vi "TestVI_TakeData.vi"() -> ()   [LabVIEW 2020]
uses:
  D:/Programs/Fatima/Lightfield-LabVIEW Automation/lightfield-automation-labview/TCube_motion/Kinesis/Thorlabs.MotionControl.Controls.dll
  Kinesis/Thorlabs.MotionControl.Controls.dll
panel:
  in  "Take data":bool
  in  "TOTAL STOP":bool
  out "Data":T1(array[cluster])
  out "ROI 1, Frame 1, Row 1":dbl[](graph)
  out "Intensity Graph":dbl[][](graph)
  in  "max":i32
  in  "min":i32
  in  "Start position X":dbl
  in  "Start position Y":dbl
  in  "Step Size Y":dbl
  in  "Step Size X":dbl
  in  "TotalSteps X":i32
  in  "TotalSteps Y":i32
  in  "SerialNumber X":string="83819717"
  in  "TCubeDCServoControl X":refnum<k24>(container)
  in  "SerialNumber Y":string="83817852"
  in  "TCubeDCServoControl Y":refnum<k24>(container)
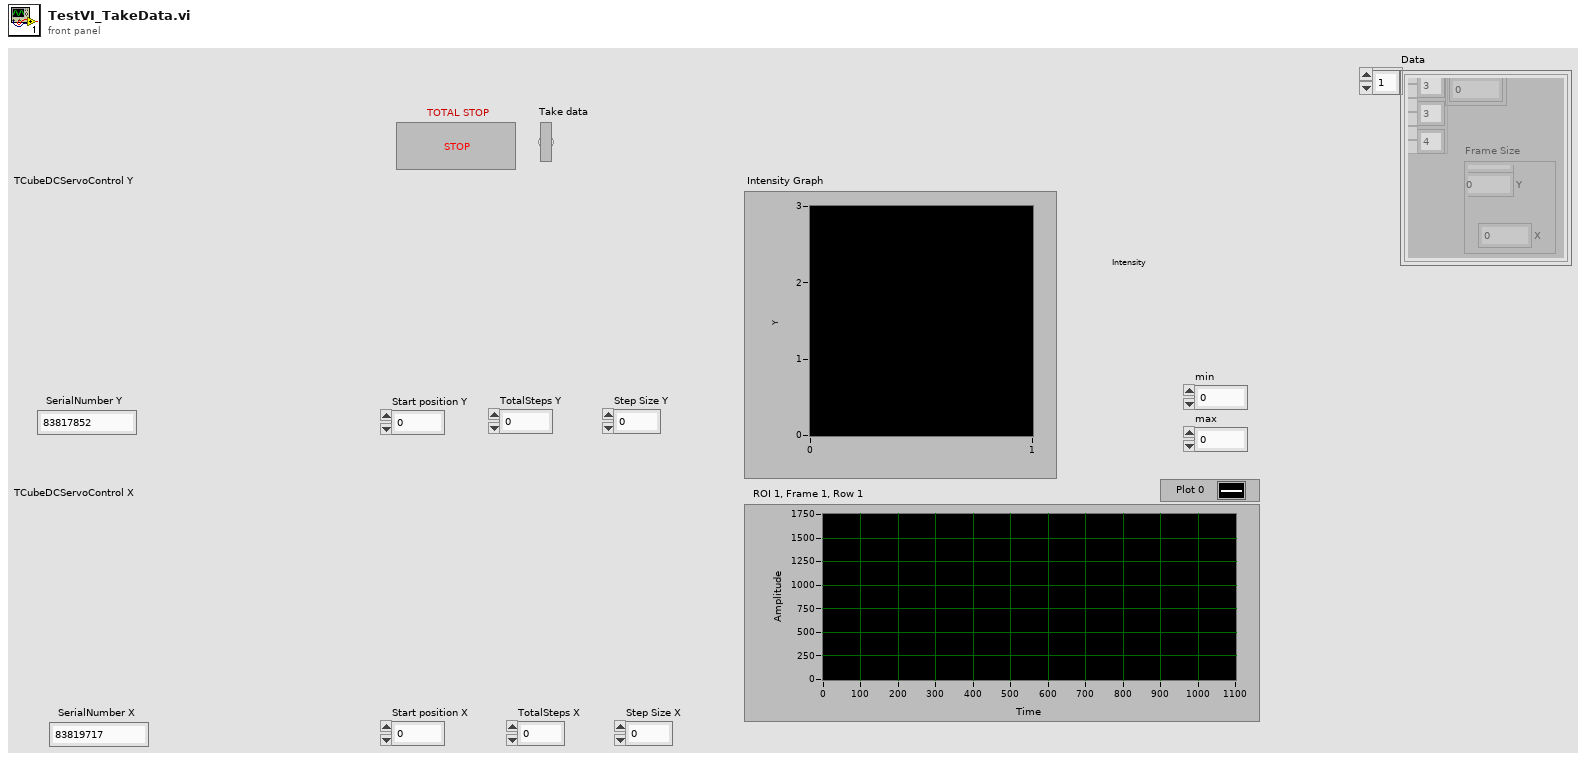
[diagram p1: front panel]
types:
  T1 = cluster{"Image":dbl[][][], "Frame Size":cluster{"F":i32, "Y":i32, "X":i32}}[]
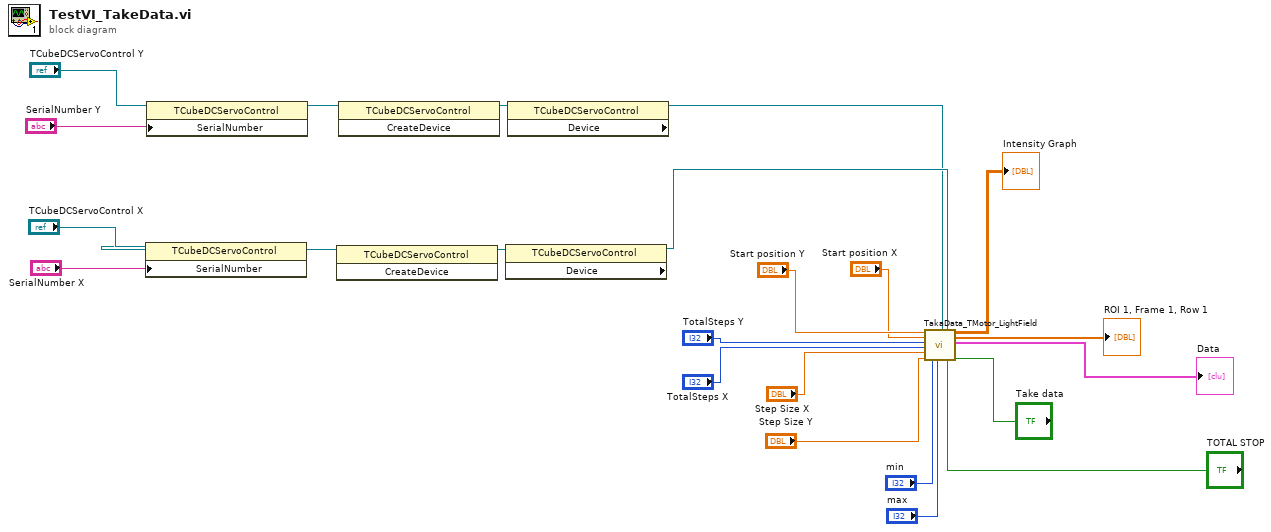
[diagram p0: block diagram]
diagram:
  n1 = property class="TCubeDCServoControl"(reference="TCubeDCServoControl X", "SerialNumber"="SerialNumber X") -> (reference out=w18:refnum<k24>)  [unwired: 1 in, 1 out]
  n2 = property class="TCubeDCServoControl"(reference="TCubeDCServoControl Y", "SerialNumber"="SerialNumber Y") -> (reference out=w19:refnum<k24>)  [unwired: 1 in, 1 out]
  n3 = invoke class="TCubeDCServoControl" method="CreateDevice"(reference=w18) -> (reference out=w17:refnum<k24>)  [unwired: 2 in, 2 out]
  n4 = invoke class="TCubeDCServoControl" method="CreateDevice"(reference=w19) -> (reference out=w16:refnum<k24>)  [unwired: 2 in, 2 out]
  n5 = property class="TCubeDCServoControl" props=["Device"](reference=w17) -> (reference out=w15:refnum<k24>)  [unwired: 1 in, 2 out]
  n6 = property class="TCubeDCServoControl" props=["Device"](reference=w16) -> (reference out=w14:refnum<k24>)  [unwired: 1 in, 2 out]
  n7 = call "TakaData_TMotor_LightField.vi"("Start position Y"="Start position Y", "Start position X"="Start position X", "TotalSteps Y"="TotalSteps Y", "TotalSteps X"="TotalSteps X", "Step Size Y"="Step Size X", "Step Size X"="Step Size Y", "min"="min", "max"="max", "TCubeDCServoControl Y"=w14, "TCubeDCServoControl X"=w15, "TOTAL STOP"="TOTAL STOP", "Take data"="Take data") -> ("Intensity Graph"=→"Intensity Graph":dbl[][], "ROI 1, Frame 1, Row 1"=→"ROI 1, Frame 1, Row 1":dbl[], "Data"=→"Data":T1)  [unwired: 5 in]
